vi "Main.vi"() -> ()   [LabVIEW 2014]
uses:
  <vilib>/DAQmx/create/channels.llb/DAQmx Create Channel (CO-Pulse Generation-Frequency).vi
  <vilib>/DAQmx/configure/timing.llb/DAQmx Timing (Implicit).vi
panel:
  in  "m2":dbl
  in  "Target RPM":dbl
  in  "t3":dbl
  in  "t2":dbl
  in  "t1":dbl
  in  "샘플링 단위(sec)":dbl
  in  "데이타 저장 경로":path
  in  "Test Unit 넘버":string
  in  "CCW":tag caption="카운터"
  in  "CW":tag caption="카운터"
  in  "Direction":bool
  in  "CW":bool
  in  "CCW":bool
  out "Voltage":dbl
  in  "Tab":enum32{"Setting", "Test"}(tab)
  in  "Test":bool
  in  "Setting":bool
  in  "Bias Check":bool
  in  "Stop":bool
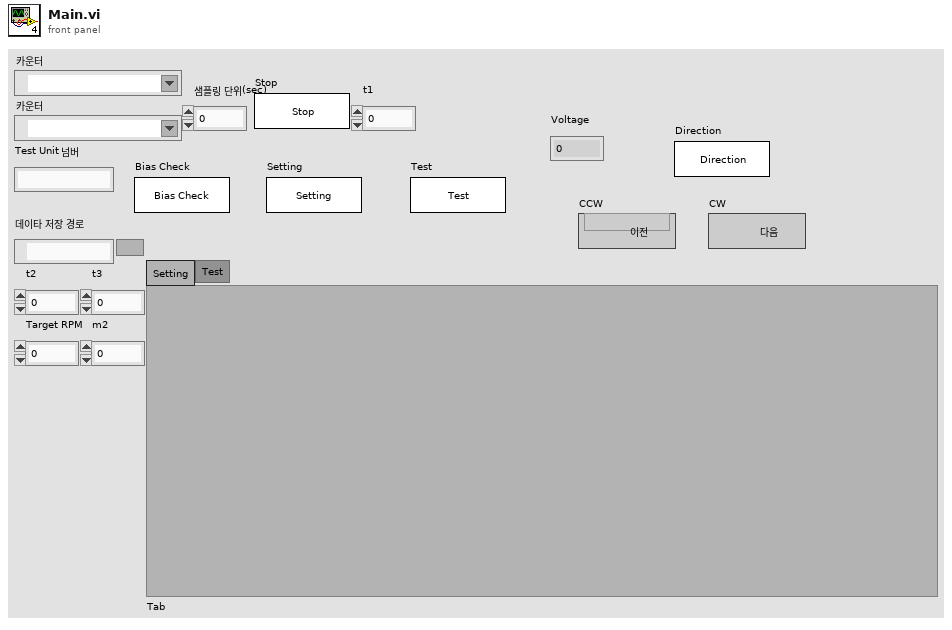
[diagram p1: front panel]
types:
  T1 = enum16{"open", "replace", "create", "open or create", "replace or create", "replace or create with confirmation"}
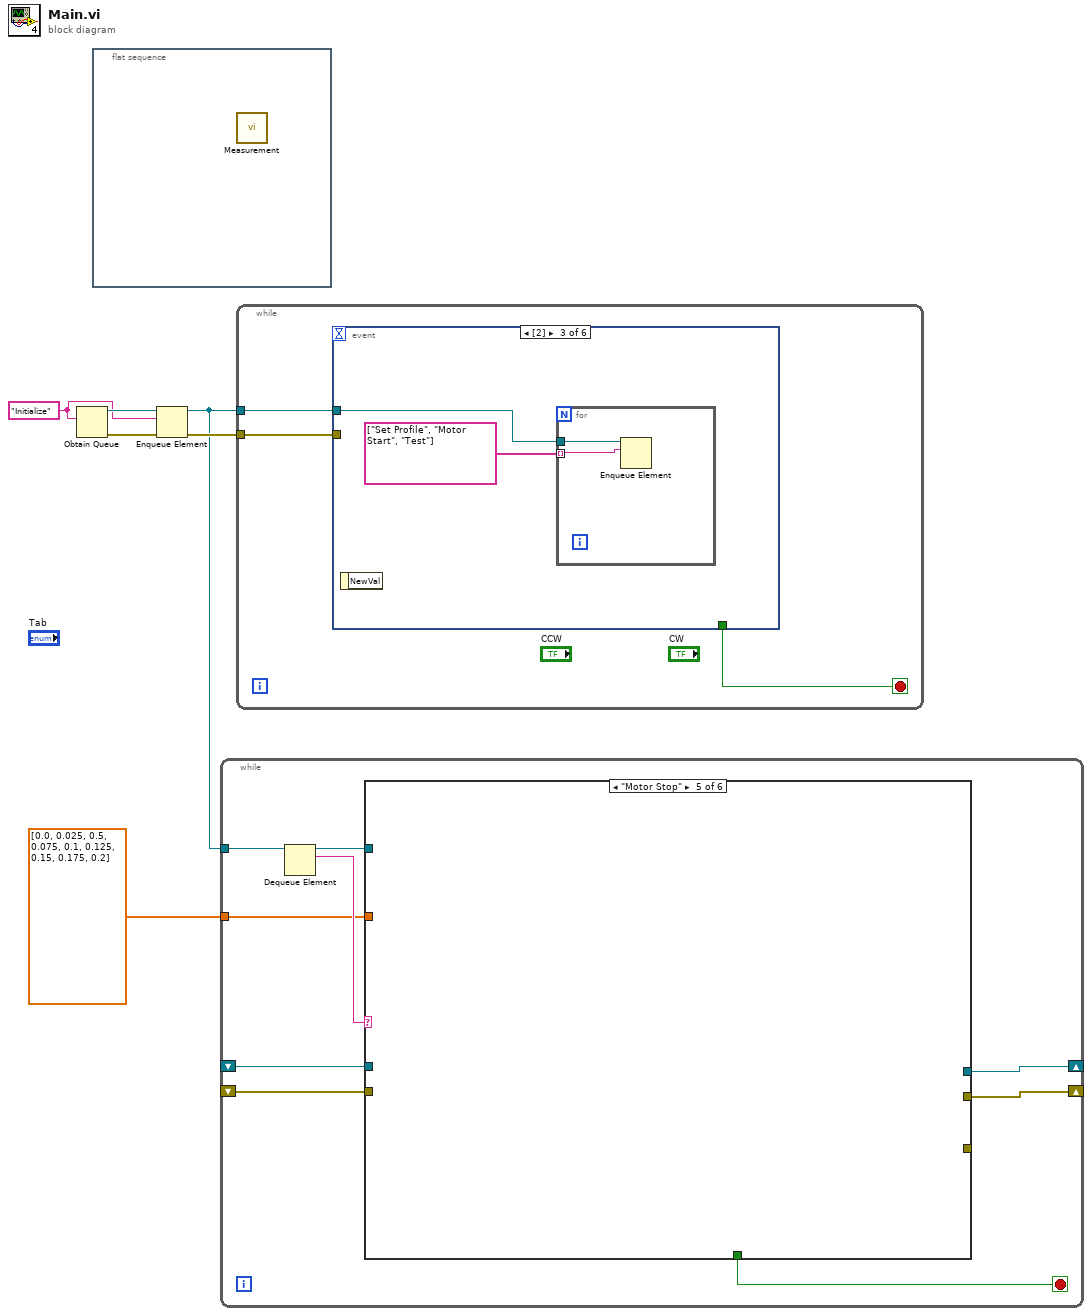
[diagram p0: block diagram]
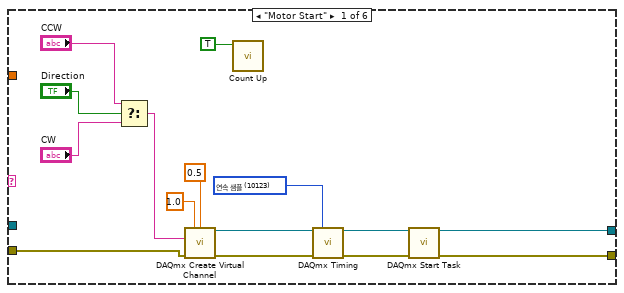
[diagram p2: hidden frame]
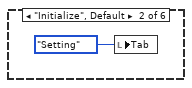
[diagram p3: hidden frame]
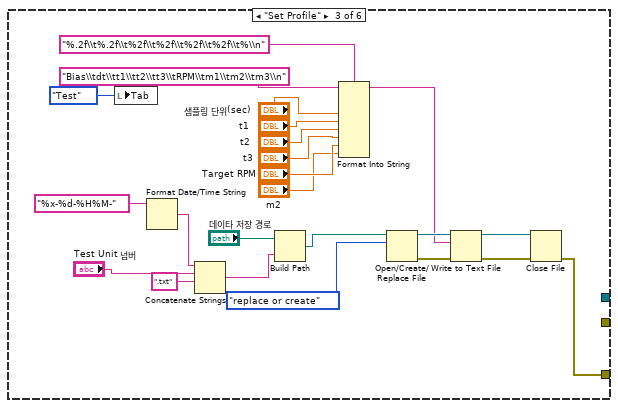
[diagram p4: hidden frame]
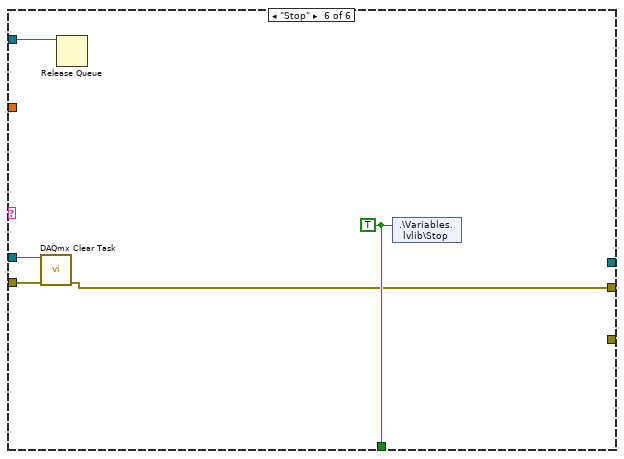
[diagram p6: hidden frame]
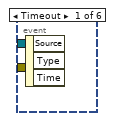
[diagram p7: hidden frame]
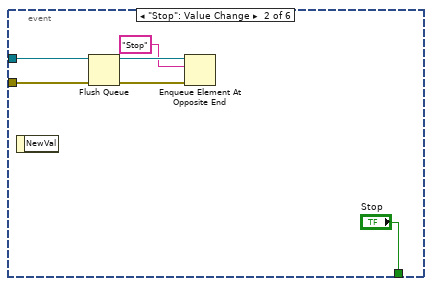
[diagram p8: hidden frame]
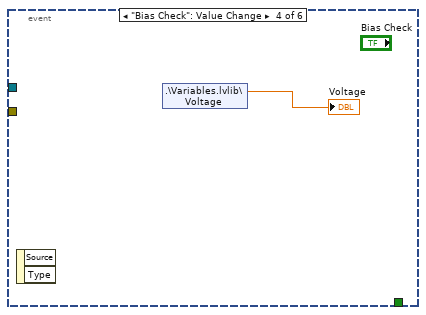
[diagram p9: hidden frame]
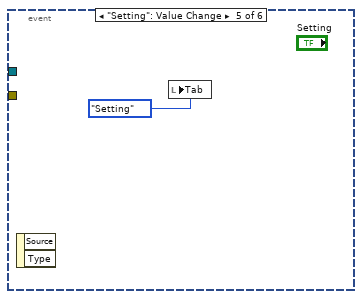
[diagram p10: hidden frame]
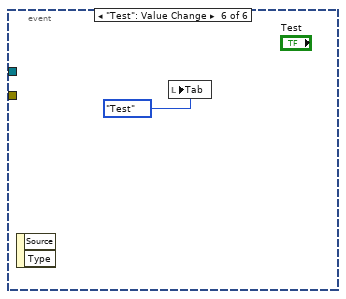
[diagram p11: hidden frame]
diagram:
  w2 = "Initialize" ("이름(이름없음)")
  n1 = Obtain Queue(element data type=w2) -> (queue out=w4:refnum<queue>, error out=w5:errorcluster)  [unwired: 4 in, 1 out]
  n2 = flat-sequence {
    frame #0 {
      n3 = call "Measurement.vi"() -> ()  [unwired: 12 in]
    }
  }
  n4 = Enqueue Element(queue=w4, element=w2, error in (no error)=w5) -> (queue out=w3:refnum<queue>, error out=w6:errorcluster)  [unwired: 1 in, 1 out]
  n5 = while {
    tunnel: w3 -> [w15]
    tunnel: dbl[] [0.0, 0.025, 0.5, 0.075, 0.1, 0.125, 0.15, 0.175, 0.2] -> [w12]
    shift-right: [w8] -> _
    shift-left: _ -> [w10]
    shift-right: [w7] -> _
    shift-left: _ -> [w9]
    stop <- w11 stop-if-true
    n6 = Dequeue Element(queue=w15) -> (queue out=w14:refnum<queue>, element=w13:string)  [unwired: 2 in, 2 out]
    n7 = case shown="\"Motor Stop\"" w13 {
      tunnel: w14 -> [_ _ _ _ _ w58]
      tunnel: w12 -> [_ _ _ _ _ _]
      tunnel: [_ _ _ _ _ w59] -> w11
      tunnel: w10 -> [_ _ _ _ _ w57]
      tunnel: w9 -> [w28 _ _ _ _ w56]
      tunnel: [w22 _ _ _ _ _] -> w8
      tunnel: [w21 _ _ _ _ w55] -> w7
      tunnel: [_ _ w43 _ _ _] -> _
      frame "Motor Start" {
        w23 = 10123 items=["유한 샘플"=10178, "연속 샘플"=10123, "하드웨어 타이밍에 의한 단일 포인트"=12522] ("sample mode")
        n8 = Select(t="CCW", s="Direction", f="CW") -> (s? t:f=w16:tag)
        n9 = call-poly <vilib>:"DAQmx Create Virtual Channel.vi"("frequency"=1.0, "duty cycle"=0.5, "counter"=w16, "error in"=w28) -> ("task out"=w27:refnum<k21>, "error out"=w26:errorcluster)  [unwired: 10 in]
        n10 = call "Count Up.vi"("Reset"=TRUE) -> ()  [unwired: 10 in, 1 out]
        n11 = call-poly <vilib>:"DAQmx Timing.vi"("task/channels in"=w27, "sample mode"=w23, "error in"=w26) -> ("task out"=w25:refnum<k21>, "error out"=w24:errorcluster)  [unwired: 11 in]
        n12 = call <vilib>:"DAQmx Start Task.vi"("task/channels in"=w25, "error in"=w24) -> ("task out"=w22:refnum<k21>, "error out"=w21:errorcluster)  [unwired: 12 in]
      }
      frame "Initialize", Default {
        n13 = local write "Tab"(enum32{"Setting", "Test"}."Setting" ("Tab")) -> ()
      }
      frame "Set Profile" {
        n14 = local write "Tab"(enum32{"Setting", "Test"}."Test" ("Tab")) -> ()
        n15 = Format Date/Time String(time format string (%c)="%x-%d-%H%M-" ("시간 포맷 문자열 (%c)")) -> (date/time string=w52:string)  [unwired: 2 in]
        n16 = Concatenate Strings(w52, "Test Unit 넘버", ".txt" ("문자열")) -> (w48:string)  [unwired: 1 in]
        n17 = Build Path(base path="데이타 저장 경로", name or relative path=w48) -> (appended path=w47:path)
        n18 = Format Into String(format string="%.2f\\t%.2f\\t%2f\\t%2f\\t%2f\\t%2f\\t%\\n" ("포맷 문자열"), initial string="Bias\\tdt\\tt1\\tt2\\tt3\\tRPM\\tm1\\tm2\\tm3\\n" ("초기 문자열"), "샘플링 단위(sec)", "t1", "t2", "t3", "Target RPM", "m2") -> (resulting string=w32:string)  [unwired: 2 in, 1 out]
        n19 = Open/Create/Replace File(file path (use dialog)=w47, operation (0:open)=T1."replace or create" ("동작(0:open)")) -> (refnum out=w42:refnum<file>, error out=w45:errorcluster)  [unwired: 4 in, 1 out]
        n20 = Write to Text File(file (use dialog)=w42, text=w32, error in=w45) -> (refnum out=w41:refnum<file>, error out=w44:errorcluster)  [unwired: 1 in, 1 out]
        n21 = Close File(refnum=w41, error in=w44) -> (error out=w43:errorcluster)  [unwired: 1 out]
      }
      frame "Test" {
      }
      frame "Motor Stop" {
      }
      frame "Stop" {
        w59 = TRUE ("Stop")
        n22 = call <vilib>:"DAQmx Clear Task.vi"("task in"=w57, "error in"=w56) -> ("error out"=w55:errorcluster)  [unwired: 13 in]
        n23 = Release Queue(queue=w58) -> ()  [unwired: 2 in, 3 out]
        n24 = shared-variable ".\\Variables.lvlib\\Stop"(w59) -> ()  [unwired: 1 in, 1 out]
      }
    }
  }
  n25 = while {
    tunnel: w3 -> [w62]
    tunnel: w6 -> [w61]
    stop <- w60 stop-if-true
    n26 = event shown="[2]" {
      selector: _ -> [_ _ _ _ _ _]
      dyn-events: _ -> [_ _ _ _ _ _]
      timeout: _ -> [_ _ _ _ _ _]
      tunnel: w62 -> [_ w68 w70 _ _ _]
      tunnel: w61 -> [_ w67 _ _ _ _]
      tunnel: [_ "Stop" _ _ _ _] -> w60
      event Timeout {
        n27 = event-data() -> ()  [unwired: 1 in, 3 out]
      }
      event "Stop": Value Change {
        n28 = event-data() -> ()  [unwired: 1 in, 1 out]
        n29 = Flush Queue(queue=w68, error in (no error)=w67) -> (queue out=w66:refnum<queue>, error out=w65:errorcluster)  [unwired: 1 out]
        n30 = Enqueue Element At Opposite End(queue=w66, element="Stop" ("이름(이름없음)"), error in (no error)=w65) -> ()  [unwired: 1 in, 3 out]
      }
      event #2 (no event record) {
        n31 = event-data() -> ()  [unwired: 1 in, 1 out]
        n32 = for {
          tunnel: w70 -> [w72]
          tunnel: string[] ["Set Profile", "Motor Start", "Test"] -> [w71] mode=indexing
          n33 = Enqueue Element(queue=w72, element=w71) -> ()  [unwired: 2 in, 3 out]
        }
      }
      event "Bias Check": Value Change {
        n34 = event-data() -> ()  [unwired: 1 in, 2 out]
        n35 = shared-variable ".\\Variables.lvlib\\Voltage"() -> (→"Voltage":dbl)  [unwired: 1 in, 1 out]
      }
      event "Setting": Value Change {
        n36 = event-data() -> ()  [unwired: 1 in, 2 out]
        n37 = local write "Tab"(enum32{"Setting", "Test"}."Setting" ("Tab")) -> ()
      }
      event "Test": Value Change {
        n38 = event-data() -> ()  [unwired: 1 in, 2 out]
        n39 = local write "Tab"(enum32{"Setting", "Test"}."Test" ("Tab")) -> ()
      }
    }
  }
